vi "KMCS2000 Record Spectrum-380nm-780nm.vi"(8 "error in (no error)":errorcluster, 11 "VISA Refnum in":refnum<visa-resource-name>) -> (0 "error out":errorcluster, 2 "Spectrum (380-780nm)":dbl[](array[numeric]), 3 "VISA Refnum out":refnum<visa-resource-name>)   [LabVIEW 2018]
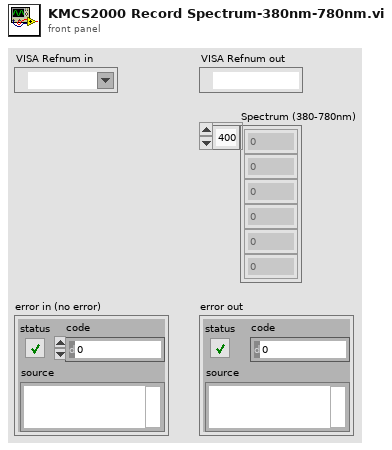
[diagram p1: front panel]
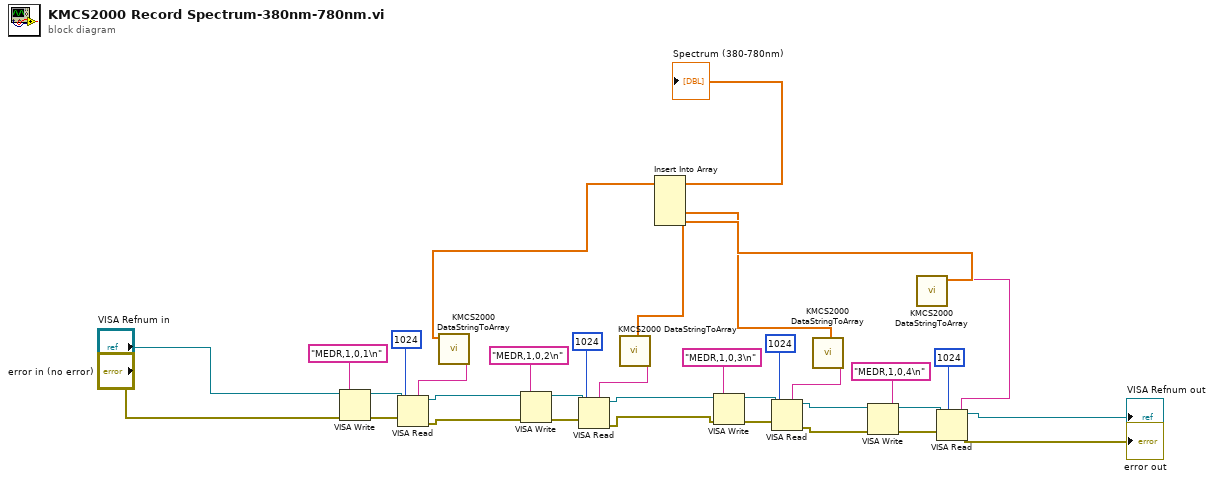
[diagram p0: block diagram]
diagram:
  n1 = VISA Write(VISA resource name="VISA Refnum in", write buffer="MEDR,1,0,1\n", error in (no error)="error in (no error)") -> (VISA resource name out=w2:refnum<visa-resource-name>, error out=w3:errorcluster)  [unwired: 1 out]
  n2 = VISA Read(VISA resource name=w2, byte count=u32 1024, error in (no error)=w3) -> (VISA resource name out=w23:refnum<visa-resource-name>, read buffer=w7:string, error out=w24:errorcluster)  [unwired: 1 out]
  n3 = call "KMCS2000 DataStringToArray.vi"("read buffer"=w7) -> ("Array"=w29:dbl[])  [unwired: 10 in]
  n4 = VISA Write(VISA resource name=w23, write buffer="MEDR,1,0,2\n", error in (no error)=w24) -> (VISA resource name out=w9:refnum<visa-resource-name>, error out=w10:errorcluster)  [unwired: 1 out]
  n5 = VISA Read(VISA resource name=w9, byte count=u32 1024, error in (no error)=w10) -> (VISA resource name out=w25:refnum<visa-resource-name>, read buffer=w12:string, error out=w26:errorcluster)  [unwired: 1 out]
  n6 = call "KMCS2000 DataStringToArray.vi"("read buffer"=w12) -> ("Array"=w30:dbl[])  [unwired: 10 in]
  n7 = VISA Write(VISA resource name=w25, write buffer="MEDR,1,0,3\n", error in (no error)=w26) -> (VISA resource name out=w14:refnum<visa-resource-name>, error out=w15:errorcluster)  [unwired: 1 out]
  n8 = VISA Read(VISA resource name=w14, byte count=u32 1024, error in (no error)=w15) -> (VISA resource name out=w27:refnum<visa-resource-name>, read buffer=w17:string, error out=w28:errorcluster)  [unwired: 1 out]
  n9 = call "KMCS2000 DataStringToArray.vi"("read buffer"=w17) -> ("Array"=w31:dbl[])  [unwired: 10 in]
  n10 = VISA Write(VISA resource name=w27, write buffer="MEDR,1,0,4\n", error in (no error)=w28) -> (VISA resource name out=w19:refnum<visa-resource-name>, error out=w20:errorcluster)  [unwired: 1 out]
  n11 = VISA Read(VISA resource name=w19, byte count=u32 1024, error in (no error)=w20) -> (VISA resource name out=→"VISA Refnum out":refnum<visa-resource-name>, read buffer=w22:string, error out=→"error out":errorcluster)  [unwired: 1 out]
  n12 = call "KMCS2000 DataStringToArray.vi"("read buffer"=w22) -> ("Array"=w32:dbl[])  [unwired: 10 in]
  n13 = Insert Into Array(array=w29, new element #1=w30, new element #2=w31, new element #3=w32) -> (→"Spectrum (380-780nm)":dbl[])  [unwired: 1 in]
